vi "Main_SideStep_GetTrace.vi"() -> ()   [LabVIEW 2020]
panel:
  in  "stop":bool
  in  "Tab Control":T1(tab)
  out "XYグラフ":T2(graph)
  in  "Select Mol Posi":u16(ring)=4 items=["3 molecules", "5 molecules", "7 molecules", "9 molecules", "13 molecules", "17 molecules", ""]
  out "Particle State":T3(array[cluster])
  in  "SD":dbl=0.11000000000000001
  in  "Tau_On":i32=40
  in  "Tau_Off":i32=10
  in  "Iteration":i32=55000
  in  "Asymmetry (X, Y)":dbl[](array[numeric])=[0.12000000000000001, 0.58]
  out "Count":i32
  in  "Torque 2":bool
  in  "Torque":dbl=-4.0
  in  "停止":bool
  in  "Rot_Noise for Cargo":bool
  in  "Width of Rot_Noise":dbl format="%#_13g"
  in  "Set_Roadblock(X, Y)":dbl[][](array[numeric])=[[30.0, -20.0], [50.0, 20.0]]
  in  "Ini_Posi (3 mol)":dbl[][](array[numeric])=[[0.0, 0.0], [6.0, 0.0], [-6.0, 0.0]]
  in  "Ini_Posi (5 mol)":dbl[][](array[numeric])=[[0.0, 0.0], [6.0, 0.0], [-6.0, 0.0], [0.0, 6.0], [0.0, -6.0]]
  in  "Ini_Posi (9 mol)":dbl[][](array[numeric])=[[0.0, 0.0], [6.0, 0.0], [-6.0, 0.0], [0.0, 6.0], [0.0, -6.0], [6.0, 6.0], [6.0, -6.0], [-6.0, 6.0], [-6.0, -6.0]]
  in  "Ini_Posi (13 mol)":dbl[][](array[numeric])=[[0.0, 0.0], [6.0, 0.0], [-6.0, 0.0], [0.0, 6.0], [0.0, -6.0], [6.0, 6.0], [6.0, -6.0], [-6.0, 6.0], [-6.0, -6.0], [3.0, 3.0], [3.0, -3.0], [-3.0, 3.0], [-3.0, -3.0]]
  in  "Ini_Posi (13 mol#2)":dbl[][](array[numeric])=[[0.0, 0.0], [12.0, 3.0], [-12.0, 3.0], [12.0, -3.0], [-12.0, -3.0], [6.0, 0.0], [-6.0, 0.0], [0.0, -6.0], [0.0, 6.0], [6.0, 6.0], [6.0, -6.0], [-6.0, 6.0], [-6.0, -6.0], [3.0, 3.0], [3.0, -3.0], [-3.0, 3.0], [-3.0, -3.0]]
  in  "Ini_Posi (7 mol)":dbl[][](array[numeric])=[[0.0, 0.0], [5.0, 3.0], [-5.0, 3.0], [5.0, -3.0], [-5.0, -3.0], [0.0, 6.0], [0.0, -6.0]]
  out "Y":dbl[](graph)
  in  "# of filaments":dbl=13.0
  out "Trajectory":cluster{"Position":dbl[], "Position":dbl[]}[](graph)
  out "Angle":dbl[](graph)
  out "Expanded Trajectory":cluster{"Position":dbl[], "Position":dbl[]}[](graph)
  in  "OK Button":bool
  # "X_Bottom, Y_Left\n\nX_Top,  Y_Right"
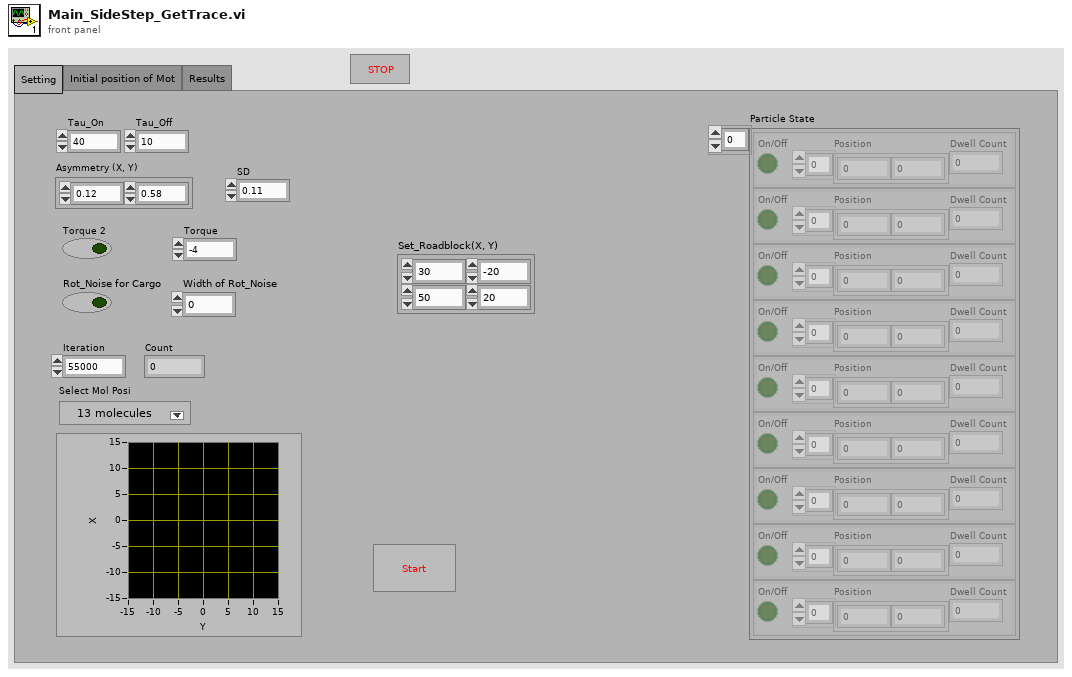
[diagram p1: front panel]
types:
  T1 = enum32{"Setting", "Initial position of Mot", "Results"}
  T2 = cluster{"Ini_Anchor_Posi (17 mol)":dbl[], "Ini_Anchor_Posi (17 mol)":dbl[]}
  T3 = cluster{"On/Off":bool, "Position":dbl[], "Dwell Count":i32}[]
  T4 = enum32{"Setting", "Initial position of Mot", "Results", "Results 2"}
  T5 = cluster{"Ini_Posi (13 mol#2)":dbl[], "Ini_Posi (13 mol#2)":dbl[]}
  T6 = cluster{"Center Position":dbl[], "Center Angle":dbl}
  T7 = cluster{"On/Off":bool, "Position":dbl[], "Next Dwell":i32}[]
  T8 = cluster{"On/Off":bool, "Position":dbl[], "Next Dwell":i32}
  T9 = enum16{"open", "replace", "create", "open or create", "replace or create", "replace or create with confirmation"}
  T10 = cluster{"Posi_Roadblock":dbl[], "Posi_Roadblock":dbl[]}
  T11 = cluster{"Posi_Roadblock":dbl[], "Posi_Roadblock":dbl[]}[]
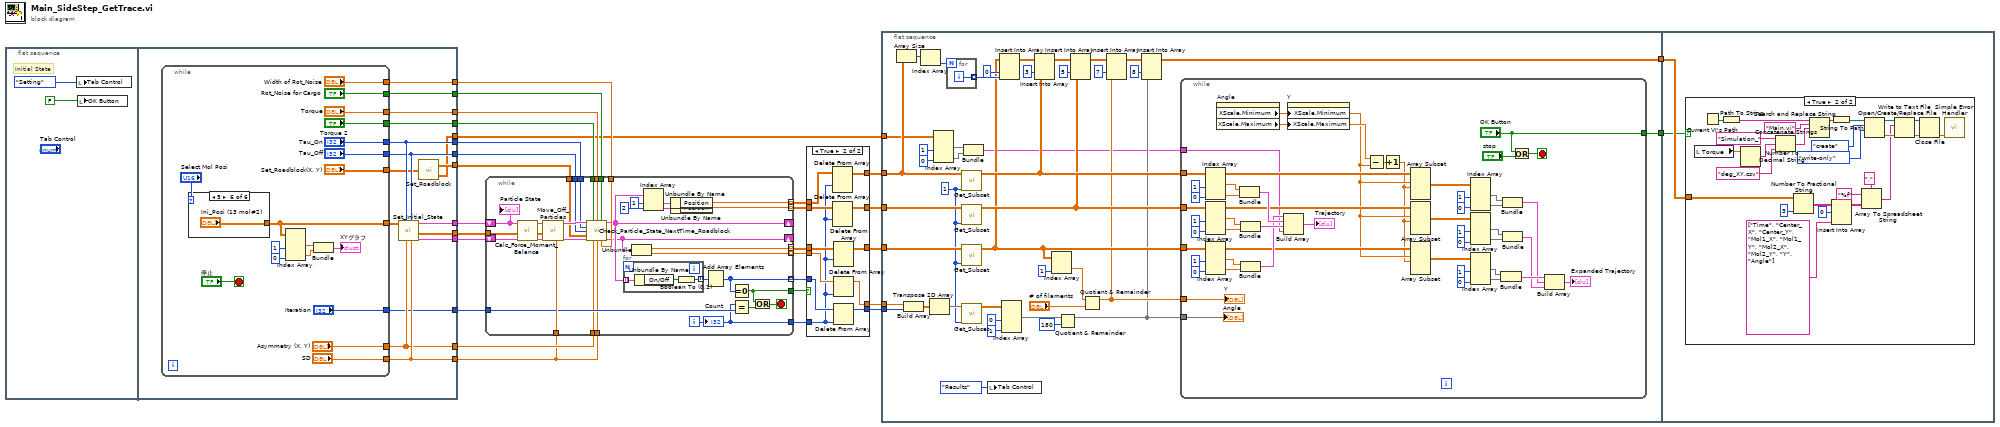
[diagram p0: block diagram]
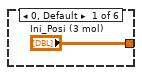
[diagram p4: hidden frame]
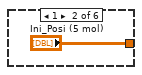
[diagram p5: hidden frame]
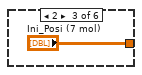
[diagram p6: hidden frame]
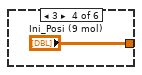
[diagram p7: hidden frame]
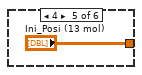
[diagram p8: hidden frame]
diagram:
  n1 = flat-sequence {
    tunnel: [w46] -> w26
    tunnel: [w45] -> w25
    tunnel: [w44] -> w24
    tunnel: [w41] -> w20
    tunnel: [w43] -> w23
    tunnel: [w42] -> w22
    tunnel: [w40] -> w21
    tunnel: [w39] -> w19
    tunnel: [w38] -> w18
    tunnel: [w36] -> w6
    tunnel: [w35] -> w5
    tunnel: [w34] -> w4
    tunnel: [w32] -> w2
    tunnel: [w31] -> w1
    frame #0 {
      # "Initial State"
      n2 = local write "Tab Control"(T4."Setting" ("Tab Control")) -> ()
      n3 = local write "OK Button"(FALSE ("OK Button")) -> ()
    }
    frame #1 {
      n4 = while {
        tunnel: ["Tau_On"] -> w43
        tunnel: ["Tau_Off"] -> w42
        tunnel: ["SD"] -> w41
        tunnel: ["Asymmetry (X, Y)"] -> w40
        tunnel: ["Torque 2"] -> w39
        tunnel: ["Torque"] -> w38
        tunnel: [w58] -> w37
        tunnel: ["Rot_Noise for Cargo"] -> w36
        tunnel: ["Width of Rot_Noise"] -> w35
        tunnel: ["Iteration"] -> w34
        tunnel: ["Set_Roadblock(X, Y)"] -> w33
        stop <- "停止" stop-if-true
        n5 = case shown="5" "Select Mol Posi" {
          tunnel: ["Ini_Posi (3 mol)" "Ini_Posi (5 mol)" "Ini_Posi (7 mol)" "Ini_Posi (9 mol)" "Ini_Posi (13 mol)" "Ini_Posi (13 mol#2)"] -> w58
          frame 0, Default {
          }
          frame 1 {
          }
          frame 2 {
          }
          frame 3 {
          }
          frame 4 {
          }
          frame 5 {
          }
        }
        n6 = Index Array(array=w58, index (col) #1=1 ("無効な指標 (列)"), index (col) #2=0 ("指標 (列)")) -> (element #1=w53:dbl[], element #2=w52:dbl[])  [unwired: 2 in]
        n7 = Bundle("Ini_Posi (13 mol#2)"=w53, "Ini_Posi (13 mol#2)"=w52) -> (→"XYグラフ":T5)  [unwired: 1 in]
      }
      n8 = call "Set_Initial_State.vi"("SD"=w41, "Tau_Off"=w42, "Asymmetry (X, Y)"=w40, "Tau_On"=w43, "Ini_Anchor_Posi"=w37) -> ("Center State at T"=w44:T6, "Ini_Anchor_Posi"=w45:dbl[][], "On_Particle State"=w46:T3)  [unwired: 4 in]
      n9 = call "Set_Roadblock.vi"("Set_Obstacles(X, Y)"=w33) -> ("Posi_Roadblock_Bound"=w32:dbl[][], "Posi_Roadblock"=w31:dbl[][])
    }
  }
  n10 = while {
    tunnel: w25 -> [w104]
    shift-right: [w71] -> _
    shift-left: w24 -> [w102]
    shift-right: [w72] -> _
    shift-left: w26 -> [w103]
    tunnel: w20 -> [w96]
    tunnel: w23 -> [w79]
    tunnel: w22 -> [w78]
    tunnel: w21 -> [w75]
    tunnel: [w99] -> w16 mode=indexing
    tunnel: [w98] -> w15 mode=indexing
    tunnel: [w97] -> w14 mode=indexing
    tunnel: w20 -> [w74]
    tunnel: w19 -> [w83]
    tunnel: w18 -> [w82]
    tunnel: [w93] -> w13 mode=indexing
    tunnel: [w88] -> w12 mode=indexing
    tunnel: w4 -> [w89]
    tunnel: [w85] -> w17
    tunnel: [w84] -> w3
    tunnel: w6 -> [w81]
    tunnel: w5 -> [w73]
    tunnel: w2 -> [w76]
    i -> [w84]
    stop <- w86 stop-if-true
    n11 = call "Calc_Force_Moment_Balance.vi"("Center State at T"=w102, "Ini_Anchor_Posi"=w104, "On_Particle State"=w103) -> ("New Center State at T"=w94:T6, "Ini_Anchor_Posi"=w95:dbl[][], "On_Particle State"=w105:T3)  [unwired: 6 in]
    n12 = call "Move_Off_Particles.vi"("SD"=w96, "Center State at T"=w94, "Ini_Anchor_Posi"=w95, "Particle Posi at T"=w105) -> ("Center State at T"=w77:T6, "New Particle Posi at T"=w80:T7)  [unwired: 6 in]
    n13 = call "Check_Particle_State_NextTime_Roadblock.vi"("Particle State at T"=w80, "Torque?"=w83, "Torque"=w82, "Rot diffusion\nfor Cargo?"=w81, "Tau_On"=w79, "Tau_Off"=w78, "Posi_Obstacles"=w76, "Center State at T"=w77, "Asymmetry (X, Y)"=w75, "SD"=w74, "Rot diffusion\nfor Cargo"=w73) -> ("Particle State at T+1"=w72:T7, "New Center State at T"=w71:T6)  [unwired: 3 in]
    n14 = for {
      tunnel: w72 -> [w108] mode=indexing
      tunnel: [w106] -> w92 mode=indexing
      n15 = Unbundle By Name(w108) -> ("On/Off"=w107:bool)
      n16 = Boolean To (0,1)(Boolean=w107) -> (0, 1=w106:i16)
    }
    n17 = Unbundle(w71) -> ("Center Position"=w97:dbl[], "Center Angle"=w93:dbl)
    n18 = Index Array(array=w72, index #1=1 ("index"), index #2=2 ("index")) -> (element #1=w101:T8, element #2=w100:T8)
    n19 = Unbundle By Name(w101) -> ("Position"=w99:dbl[])
    n20 = Unbundle By Name(w100) -> ("Position"=w98:dbl[])
    n21 = Add Array Elements(numeric array=w92) -> (sum=w88:i16)
    n22 = Equal To 0?(x=w88) -> (x = 0?=w85:bool)
    n23 = Equal?(x=w84, y=w89) -> (x = y?=w87:bool)
    n24 = Or(x=w85, y=w87) -> (x .or. y?=w86:bool)
    "Particle State" <- w103
    "Count" <- w84
  }
  n25 = case shown="TRUE" w17 {
    tunnel: w16 -> [w113 w124]
    tunnel: w15 -> [w112 w123]
    tunnel: w3 -> [_ w119]
    tunnel: w14 -> [w111 w122]
    tunnel: w13 -> [w110 w121]
    tunnel: w12 -> [w109 w120]
    tunnel: [w109 w118] -> w11
    tunnel: [w110 w117] -> w10
    tunnel: [w111 w116] -> w9
    tunnel: [w112 w115] -> w8
    tunnel: [w113 w114] -> w7
    frame False {
    }
    frame True {
      n26 = Delete From Array(array=w124, index (row)=w119) -> (array with subset deleted=w114:dbl[][])  [unwired: 2 in, 1 out]
      n27 = Delete From Array(array=w123, index (row)=w119) -> (array with subset deleted=w115:dbl[][])  [unwired: 2 in, 1 out]
      n28 = Delete From Array(array=w122, index (row)=w119) -> (array with subset deleted=w116:dbl[][])  [unwired: 2 in, 1 out]
      n29 = Delete From Array(array=w121, index=w119) -> (array with subset deleted=w117:dbl[])  [unwired: 1 in, 1 out]
      n30 = Delete From Array(array=w120, index=w119) -> (array with subset deleted=w118:i16[])  [unwired: 1 in, 1 out]
    }
  }
  n31 = flat-sequence {
    tunnel: w7 -> [w133]
    tunnel: w8 -> [w166]
    tunnel: w9 -> [w165]
    tunnel: w10 -> [w164]
    tunnel: w11 -> [w158]
    tunnel: [w138] -> w28
    tunnel: [w155] -> w27
    tunnel: w1 -> [w130]
    tunnel: w28 -> [w217]
    tunnel: w27 -> [w216]
    frame #0 {
      w134 = 1
      n32 = Array Size(array=w133) -> (size(s)=w132:i32[])
      n33 = Build Array(w164, w158) -> (w163:dbl[][])
      n34 = Index Array(array=w132) -> (element=w131:i32)  [unwired: 1 in]
      n35 = Transpose 2D Array(2D array=w163) -> (transposed array=w162:dbl[][])
      n36 = Index Array(array=w130, index (col) #1=1 ("無効な指標 (列)"), index (col) #2=0 ("指標 (列)")) -> (element #1=w127:dbl[], element #2=w126:dbl[])  [unwired: 2 in]
      n37 = for {
        N: w131 -> [_]
        tunnel: [w167] -> w157 mode=indexing
        i -> [w167]
      }
      n38 = call "Get_Subset.vi"("index"=w134, "Input"=w133) -> ("Output"=w153:dbl[][])  [unwired: 9 in]
      n39 = call "Get_Subset.vi"("index"=w134, "Input"=w166) -> ("Output"=w150:dbl[][])  [unwired: 9 in]
      n40 = call "Get_Subset.vi"("index"=w134, "Input"=w165) -> ("Output"=w146:dbl[][])  [unwired: 9 in]
      n41 = call "Get_Subset.vi"("index"=w134, "Input"=w162) -> ("Output"=w161:dbl[][])  [unwired: 9 in]
      n42 = Bundle("Posi_Roadblock"=w127, "Posi_Roadblock"=w126) -> (w125:T10)  [unwired: 1 in]
      n43 = local write "Tab Control"(T4."Results" ("Tab Control")) -> ()
      n44 = Insert Into Array(array=w146, index (col)=0 ("disabled index (col)"), new element=w157) -> (w154:dbl[][])  [unwired: 1 in]
      n45 = Index Array(array=w161, index (col) #1=0 ("disabled index (col)"), index (col) #2=1 ("index (col)")) -> (element #1=w147:dbl[])  [unwired: 2 in, 1 out]
      n46 = Insert Into Array(array=w154, index (col)=3 ("disabled index (col)"), new element=w153) -> (w151:dbl[][])  [unwired: 1 in]
      n47 = Index Array(array=w146, index (col)=1 ("disabled index (col)")) -> (element=w144:dbl[])  [unwired: 1 in]
      n48 = Quotient & Remainder(x=w147, y=180) -> (x-y*floor(x/y)=w137:dbl[])  [unwired: 1 out]
      n49 = Insert Into Array(array=w151, index (col)=5 ("disabled index (col)"), new element=w150) -> (w142:dbl[][])  [unwired: 1 in]
      n50 = Quotient & Remainder(x=w144, y="# of filaments") -> (x-y*floor(x/y)=w141:dbl[])  [unwired: 1 out]
      n51 = Insert Into Array(array=w142, index (col)=7 ("disabled index (col)"), new element=w141) -> (w139:dbl[][])  [unwired: 1 in]
      n52 = Insert Into Array(array=w139, index (col)=8 ("disabled index (col)"), new element=w137) -> (w138:dbl[][])  [unwired: 1 in]
      n53 = while {
        tunnel: w153 -> [w201]
        tunnel: w150 -> [w198]
        tunnel: w146 -> [w197]
        tunnel: ["OK Button"] -> w155
        tunnel: w137 -> [w169]
        tunnel: w141 -> [w170]
        tunnel: w125 -> [w168]
        stop <- w173 stop-if-true
        n54 = Index Array(array=w201, index (col) #1=1 ("disabled index (col)"), index (col) #2=0 ("index (col)")) -> (element #1=w202:dbl[], element #2=w211:dbl[])  [unwired: 2 in]
        n55 = Index Array(array=w198, index (col) #1=1 ("disabled index (col)"), index (col) #2=0 ("index (col)")) -> (element #1=w203:dbl[], element #2=w210:dbl[])  [unwired: 2 in]
        n56 = Index Array(array=w197, index (col) #1=1 ("disabled index (col)"), index (col) #2=0 ("index (col)")) -> (element #1=w171:dbl[], element #2=w205:dbl[])  [unwired: 2 in]
        n57 = property on="Angle" class="WFGraph (指定)"() -> ("XScale.Minimum"=w176:dbl, "XScale.Maximum"=w200:dbl)  [unwired: 2 in, 2 out]
        n58 = Bundle("Output"=w202, "Output"=w211) -> (w209:cluster{"Output":dbl[], "Output":dbl[]})  [unwired: 1 in]
        n59 = Bundle("Output"=w203, "Output"=w210) -> (w208:cluster{"Output":dbl[], "Output":dbl[]})  [unwired: 1 in]
        n60 = Bundle("Output"=w171, "Output"=w205) -> (w204:cluster{"Output":dbl[], "Output":dbl[]})  [unwired: 1 in]
        n61 = Build Array(w204, w209, w208, w168) -> (→"Trajectory":T11)
        n62 = property on="Y" class="WFGraph (指定)"("XScale.Minimum"=w176, "XScale.Maximum"=w200) -> ()  [unwired: 2 in, 2 out]
        n63 = Subtract(x=w200, y=w176) -> (x-y=w199:dbl)
        n64 = Increment(x=w199) -> (x+1=w175:dbl)
        n65 = Array Subset(array=w201, index (row)=w176, length (row)=w175) -> (w178:dbl[][])  [unwired: 2 in]
        n66 = Array Subset(array=w198, index (row)=w176, length (row)=w175) -> (w177:dbl[][])  [unwired: 2 in]
        n67 = Array Subset(array=w197, index (row)=w176, length (row)=w175) -> (w179:dbl[][])  [unwired: 2 in]
        n68 = Index Array(array=w178, index (col) #1=1 ("disabled index (col)"), index (col) #2=0 ("index (col)")) -> (element #1=w190:dbl[], element #2=w189:dbl[])  [unwired: 2 in]
        n69 = Index Array(array=w177, index (col) #1=1 ("disabled index (col)"), index (col) #2=0 ("index (col)")) -> (element #1=w188:dbl[], element #2=w187:dbl[])  [unwired: 2 in]
        n70 = Index Array(array=w179, index (col) #1=1 ("disabled index (col)"), index (col) #2=0 ("index (col)")) -> (element #1=w186:dbl[], element #2=w185:dbl[])  [unwired: 2 in]
        n71 = Bundle(w186, w185) -> (w184:cluster{dbl[], dbl[]})  [unwired: 1 in]
        n72 = Bundle(w190, w189) -> (w183:cluster{dbl[], dbl[]})  [unwired: 1 in]
        n73 = Bundle(w188, w187) -> (w182:cluster{dbl[], dbl[]})  [unwired: 1 in]
        n74 = Or(x="OK Button", y="stop") -> (x .or. y?=w173:bool)
        n75 = Build Array(w184, w183, w182) -> (→"Expanded Trajectory":cluster{dbl[], dbl[]}[])
        "Angle" <- w169
        "Y" <- w170
      }
    }
    frame #1 {
      n76 = case shown="TRUE" w216 {
        tunnel: w217 -> [_ w227]
        frame False {
        }
        frame True {
          n77 = local read "Torque"() -> (w226:dbl)
          n78 = Current VI's Path() -> (path=w222:path)
          n79 = Path To String(path=w222) -> (string=w221:string)
          n80 = Number To Decimal String(number=w226) -> (decimal integer string=w224:string)  [unwired: 1 in]
          n81 = Concatenate Strings("Simulation_" ("文字列"), w224, "deg_XY.csv" ("string")) -> (w219:string)
          n82 = Number To Fractional String(number=w227, precision (6)=i16 3) -> (F-format string=w235:string[][])  [unwired: 2 in]
          n83 = Search and Replace String(input string=w221, search string="Main.vi", replace string=w219) -> (result string=w218:string)  [unwired: 5 in, 3 out]
          n84 = String To Path(string=w218) -> (path=w236:path)
          n85 = Insert Into Array(array=w235, index (row)=0, new element=string[] ["Time", "Center_X", "Center_Y", "Mol1_X", "Mol1_Y", "Mol2_X", "Mol2_Y", "Y", "Angle"]) -> (w233:string[][])  [unwired: 1 in]
          n86 = Array To Spreadsheet String(delimiter (Tab)=",", array=w233, 3:"%f" ("format string")) -> (spreadsheet string=w231:string)
          n87 = Open/Create/Replace File(file path (use dialog)=w236, operation (0:open)=T9."create", access (0:read/write)=enum16{"read/write", "read-only", "write-only"}."write-only") -> (refnum out=w239:refnum<file>, error out=w240:errorcluster)  [unwired: 1 in, 3 out]
          n88 = Write to Text File(file (use dialog)=w239, text=w231, error in=w240) -> (refnum out=w242:refnum<file>, error out=w243:errorcluster)  [unwired: 1 in, 1 out]
          n89 = Close File(refnum=w242, error in=w243) -> (error out=w241:errorcluster)  [unwired: 1 out]
          n90 = call <vilib>:"Simple Error Handler.vi"("error in (no error)"=w241) -> ()  [unwired: 1 in, 8 out]
        }
      }
    }
  }
